vi "Brake On.vi"(8 "error in (no error)":errorcluster, 11 "Comp Motors with Brake in":refnum<class "Comp Motors with Brake.lvclass">) -> (0 "error out":errorcluster, 3 "Comp Motors with Brake out":refnum<class "Comp Motors with Brake.lvclass">)   [LabVIEW 2014, in "Comp Motors with Brake.lvlib" / "Comp Motors with Brake.lvclass"]
uses:
  Comp Motors with Brake.lvclass
  <vilib>/Rock Robotics/WPI/Solenoid/WPI_SolenoidValue.ctl
  Comp Motors with Brake.lvclass/Comp Motors with Brake.ctl
  <vilib>/Rock Robotics/WPI/Solenoid/WPI_SolenoidSetEnum.vi
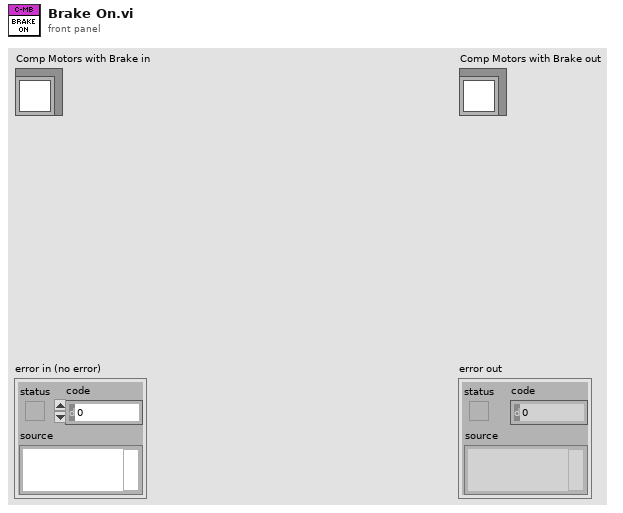
[diagram p1: front panel]
types:
  T1 = typedef "WPI_SolenoidValue.ctl" = enum16{"Off", "On", "Forward", "Reverse"}
  T2 = typedef "WPI_SolenoidDevRef.ctl" = cluster{"DevStatus":errorcluster, "Pneumatics Control Module":u8, "Forward Solenoid Channel":T3, "Reverse Solenoid Channel":T3}
  T3 = typedef "WPI_SolenoidChannel.ctl" = enum8{"Solenoid 0", "Solenoid 1", "Solenoid 2", "Solenoid 3", "Solenoid 4", "Solenoid 5", "Solenoid 6", "Solenoid 7", "Invalid"}
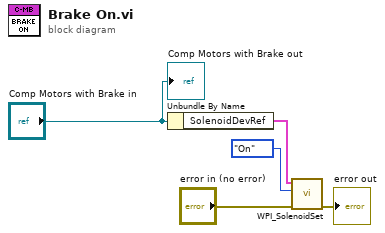
[diagram p0: block diagram]
diagram:
  n1 = Unbundle By Name("Comp Motors with Brake in") -> ("SolenoidDevRef"=w4:T2)
  n2 = call-poly <vilib>:"WPI_SolenoidSet.vi"("error in (no error)"="error in (no error)", "Value"=WPI_SolenoidValue."On", "SolenoidDevRef"=w4) -> ("error out"=→"error out":errorcluster)  [unwired: 7 in, 1 out]
  "Comp Motors with Brake out" <- "Comp Motors with Brake in"
